vi "Graphics-Sort XY Graph (1D).vi"(7 "graph":cluster{"x":dbl[], "y":dbl[]}[](array[cluster])) -> (8 "sorted graph":cluster{"x":dbl[], "y":dbl[]}[](array[cluster]))   [LabVIEW 2020]
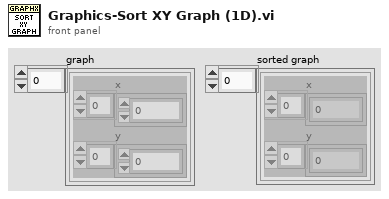
[diagram p1: front panel]
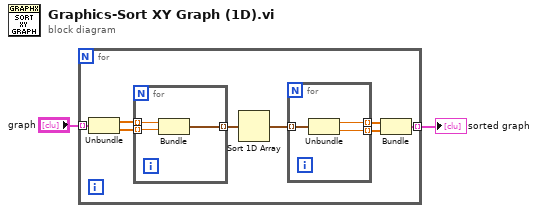
[diagram p0: block diagram]
diagram:
  n1 = for {
    tunnel: "graph" -> [w9] mode=indexing
    tunnel: [w3] -> w1 mode=indexing
    n2 = Unbundle(w9) -> ("x"=w8:dbl[], "y"=w7:dbl[])
    n3 = for {
      tunnel: w8 -> [w16] mode=indexing
      tunnel: [w15] -> w10 mode=indexing
      tunnel: w7 -> [w14] mode=indexing
      n4 = Bundle("Numeric"=w16, "Numeric"=w14) -> (w15:cluster{"Numeric":dbl, "Numeric":dbl})  [unwired: 1 in]
    }
    n5 = Sort 1D Array(array=w10) -> (sorted array=w6:cluster{"Numeric":dbl, "Numeric":dbl}[])
    n6 = for {
      tunnel: w6 -> [w13] mode=indexing
      tunnel: [w12] -> w5 mode=indexing
      tunnel: [w11] -> w4 mode=indexing
      n7 = Unbundle(w13) -> ("Numeric"=w12:dbl, "Numeric"=w11:dbl)
    }
    n8 = Bundle(w5, w4) -> (w3:cluster{dbl[], dbl[]})  [unwired: 1 in]
  }
  "sorted graph" <- w1
